vi "Get ctrl Primary Button.vi"(3 "Button Primary":T1) -> (0 "Button Primary":bool)   [LabVIEW 2014]
uses:
  Button Actions.ctl
  SRE Enum.ctl
  Support Code/Robot Global Data.vi
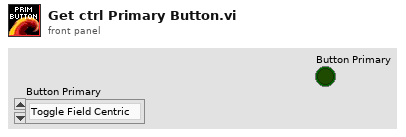
[diagram p1: front panel]
types:
  T1 = typedef "Button Actions.ctl" = enum16{"Toggle Field Centric", "Gyro Reset", "Clear Faults", "Reduce Speed"}
  T2 = enum16{"Trigger Left", "2 Left", "3 Left", "4 Left", "5 Left", "6 Left", "7 Left", "8 Left", "9 Left", "10 Left", "11 Left", "Trigger Right", "2 Right", "3 Right", "4 Right", "5 Right", "6 Right", "7 Right", "8 Right", "9 Right", "10 Right", "11 Right"}[]
  T3 = typedef "SRE Enum.ctl" = enum16{"Start", "Run", "End"}
  T4 = enum16{"Trigger Left", "2 Left", "3 Left", "4 Left", "5 Left", "6 Left", "7 Left", "8 Left", "9 Left", "10 Left", "11 Left", "Trigger Right", "2 Right", "3 Right", "4 Right", "5 Right", "6 Right", "7 Right", "8 Right", "9 Right", "10 Right", "11 Right"}
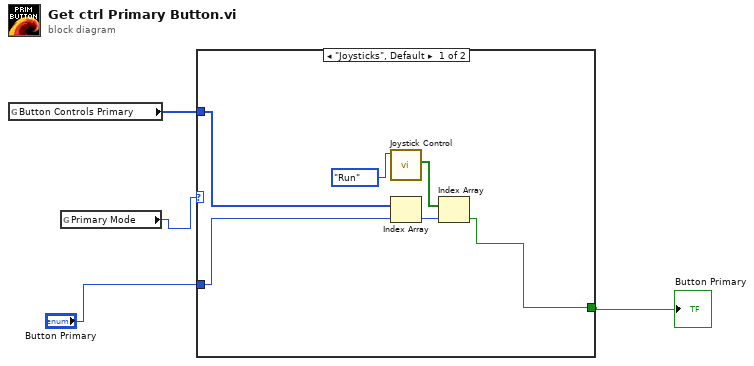
[diagram p0: block diagram]
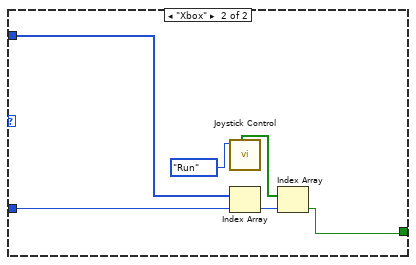
[diagram p2: hidden frame]
diagram:
  n1 = global read "Robot Global Data.vi" "Button Controls Primary"() -> (w2:T2)
  n2 = global read "Robot Global Data.vi" "Primary Mode"() -> (w4:enum16{"Joysticks", "Xbox"})
  n3 = case shown="\"Joysticks\", Default" w4 {
    tunnel: "Button Primary" -> [w7 w13]
    tunnel: [w6 w12] -> w1
    tunnel: w2 -> [w8 w11]
    frame "Joysticks", Default {
      n4 = call "Joystick Control.vi"("Enum"=SRE_Enum."Run") -> ("Button Output PJ"=w5:bool[])  [unwired: 3 in, 5 out]
      n5 = Index Array(array=w8, index=w7) -> (element=w9:T4)
      n6 = Index Array(array=w5, index=w9) -> (element=w6:bool)
    }
    frame "Xbox" {
      n7 = call "Joystick Control.vi"("Enum"=SRE_Enum."Run") -> ("Buttons Output PX"=w14:bool[])  [unwired: 3 in, 5 out]
      n8 = Index Array(array=w11, index=w13) -> (element=w15:T4)
      n9 = Index Array(array=w14, index=w15) -> (element=w12:bool)
    }
  }
  "Button Primary" <- w1
